vi "Create Pipeline.vi"(11 "Array in":refnum<class "Message Enqueuer.lvclass">[](array[class])) -> (1 "Last":refnum<class "Message Enqueuer.lvclass">, 2 "First":refnum<class "Message Enqueuer.lvclass">, 3 "Array out":refnum<class "Message Enqueuer.lvclass">[](array[class]))   [LabVIEW 2014, in "Pipelined Actor.lvlib" / "Pipelined Actor.lvclass"]
uses:
  Pipelined Actor.lvclass
  <vilib>/ActorFramework/Message Enqueuer/Message Enqueuer.lvclass
  Pipelined Actor Messages/Set Next Actor Msg/Set Next Actor Msg.lvclass/Set Next Actor Msg.ctl
  <vilib>/ActorFramework/Message Enqueuer/Message Enqueuer.lvclass/Message Enqueuer.ctl
  <vilib>/ActorFramework/Message Enqueuer/Enqueue.vi
  <vilib>/ActorFramework/Message Priority Queue/Priority Enqueue.vi
  Pipelined Actor Messages/Set Next Actor Msg/Set Next Actor Msg.lvclass
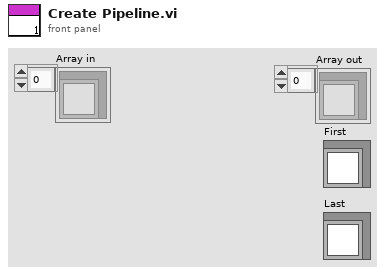
[diagram p1: front panel]
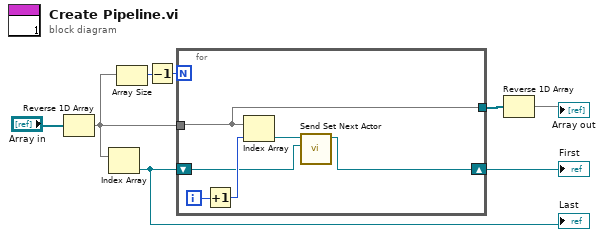
[diagram p0: block diagram]
diagram:
  n1 = Reverse 1D Array(array="Array in") -> (reversed array=w4:refnum<class "Message Enqueuer.lvclass">[])
  n2 = Index Array(array=w4) -> (element=w6:refnum<class "Message Enqueuer.lvclass">)  [unwired: 1 in]
  "Last" <- w6
  n3 = Array Size(array=w4) -> (size(s)=w3:i32)
  n4 = Decrement(x=w3) -> (x-1=w2:i32)
  n5 = for {
    N: w2 -> [_]
    tunnel: w4 -> [w12]
    shift-right: [w9] -> w7
    shift-left: w6 -> [w10]
    tunnel: [w12] -> w5
    i -> [w14]
    n6 = Increment(x=w14) -> (x+1=w13:i32)
    n7 = Index Array(array=w12, index=w13) -> (element=w11:refnum<class "Message Enqueuer.lvclass">)
    n8 = call "Send Set Next Actor.vi"("Next Pipelined Actor"=w10, "Message Enqueuer"=w11) -> ("Message Enqueuer out"=w9:refnum<class "Message Enqueuer.lvclass">)  [unwired: 8 in, 1 out]
  }
  "First" <- w7
  n9 = Reverse 1D Array(array=w5) -> (reversed array=→"Array out":refnum<class "Message Enqueuer.lvclass">[])
